vi "Get GUI reference.vi"(8 "error in (no error)":errorcluster, 11 "Scan SBlock in":refnum<class "Scan SBlock.lvclass">) -> (0 "error out":errorcluster, 2 "reference out":refnum<vi>, 3 "Scan SBlock out":refnum<class "Scan SBlock.lvclass">)   [LabVIEW 2020, in "CIRCUS_uServices.lvlib" / "Run Utilities.lvlib" / "Scan SBlock.lvclass"]
doc: "Create a GUI element for this SBlock"
uses:
  Scan SBlock.lvclass
  Advanced Parameters - list.ctl
  Advanced Panel Parameter Mode.ctl
  Advanced Parameters.ctl
panel:
  out "Parameters from List":T1[](array[typedef])
  out "Parameters from Steps":T2[](array[typedef]) caption="Parameters from Steps                  From    To              Step           Mode"
  out "No. of linked \nsteps":u32
  out "Common Parameters":string[][](array[string])
  out "Kasli":string
  out "Number of repetitions":u16=1 min=1
  out "Script name":string
  # "Parameters from lists"
  # "List of values"
  # "Parameters from steps"
  # "From"
  # "To"
  # "Step size"
  # "Mode"
  # "Parameter Name"
  # "Parameter Value"
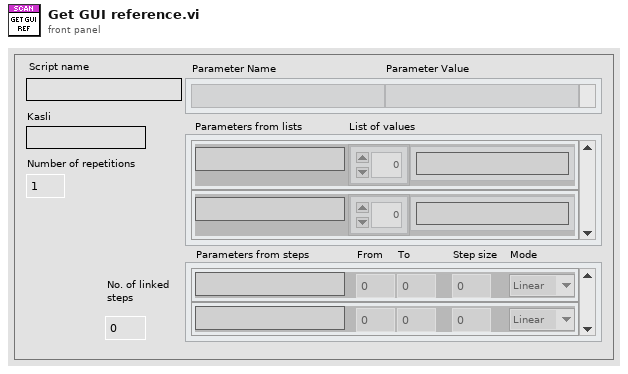
[diagram p1: front panel]
types:
  T1 = typedef "CIRCUS_uServices.lvlib/Run Utilities.lvlib/Scan SBlock.lvclass/Advanced Parameters - list.ctl" = cluster{"Param":string, "List of values":string[]}
  T2 = typedef "CIRCUS_uServices.lvlib/Run Utilities.lvlib/Scan SBlock.lvclass/Advanced Parameters.ctl" = cluster{"Param":string, "From":dbl, "To":dbl, "Step":dbl, "Mode":T3}
  T3 = typedef "CIRCUS_uServices.lvlib/Run Utilities.lvlib/Scan SBlock.lvclass/Advanced Panel Parameter Mode.ctl" = enum16{"Linear", "Log", "LINKED"}
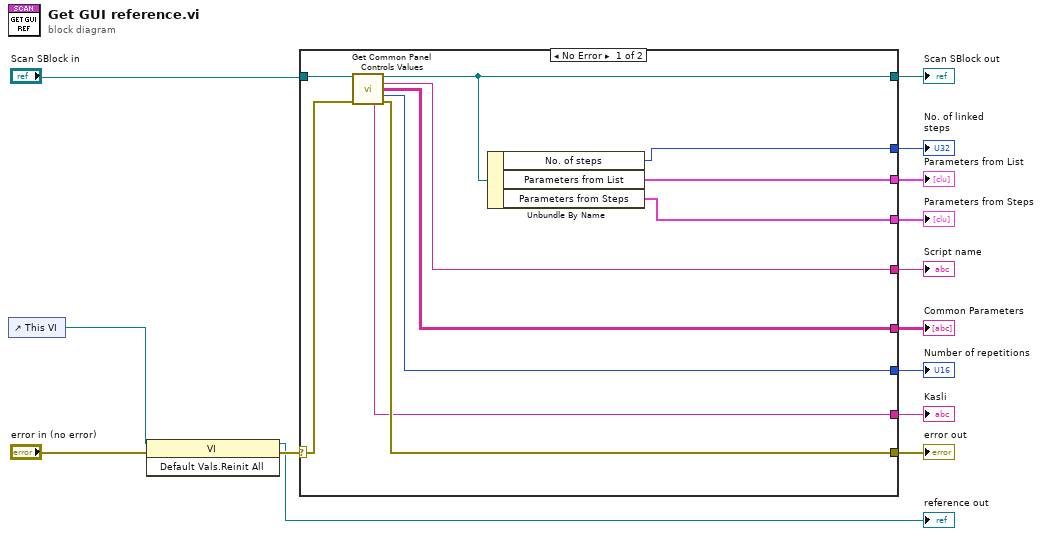
[diagram p0: block diagram]
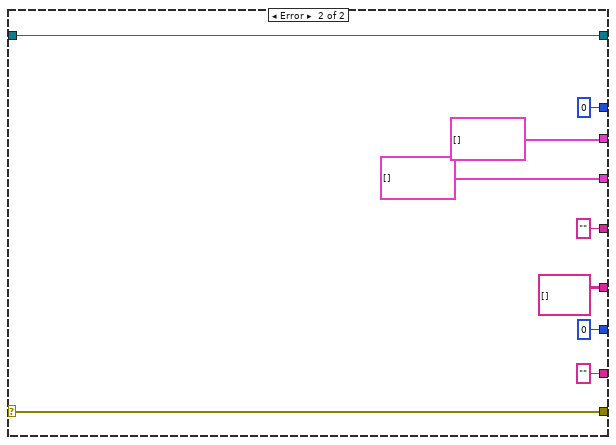
[diagram p2: hidden frame]
diagram:
  n1 = control-ref of="This VI"() -> (w13:refnum<vi>)
  n2 = invoke class="VI" method="Default Vals.Reinit All"(reference=w13, error in="error in (no error)") -> (reference out=→"reference out":refnum<vi>, error out=w11:errorcluster)  [unwired: 1 in, 1 out]
  n3 = case shown="No Error" w11 {
    selector: w11 -> [w24 w34]
    tunnel: [w23 w34] -> w9
    tunnel: [w18 w33] -> w8
    tunnel: "Scan SBlock in" -> [w25 w33]
    tunnel: [w22 "" ("Kasli Name")] -> w7
    tunnel: [w21 u16 0 ("Number of repetitions")] -> w6
    tunnel: [w20 string[][] [] ("Common Parameters")] -> w5
    tunnel: [w19 "" ("Script Name")] -> w4
    tunnel: [w17 u32 0 ("No. of steps")] -> w3
    tunnel: [w16 T1[] [] ("Parameters from List")] -> w2
    tunnel: [w15 T2[] [] ("Parameters from Steps")] -> w1
    frame No Error {
      n4 = call-dynamic "Get Common Panel Controls Values.vi"("Schedule Block in"=w25, "error in (no error)"=w24) -> ("Schedule Block out"=w18:refnum<class "Scan SBlock.lvclass">, "Script Name"=w19:string, "Common Parameters"=w20:string[][], "Number of repetitions"=w21:u16, "FPGA Name"=w22:string, "error out"=w23:errorcluster)  [unwired: 7 in, 1 out]
      n5 = Unbundle By Name(w18) -> ("No. of steps"=w17:u32, "Parameters from List"=w16:T1[], "Parameters from Steps"=w15:T2[])
    }
    frame Error {
    }
  }
  "error out" <- w9
  "Scan SBlock out" <- w8
  "Script name" <- w4
  "Number of repetitions" <- w6
  "Common Parameters" <- w5
  "Kasli" <- w7
  "No. of linked \nsteps" <- w3
  "Parameters from Steps" <- w1
  "Parameters from List" <- w2
